vi "Write.vi"(8 "error in (no error)":errorcluster, 10 "Value":sgl, 11 "Local Bus_DBL in":refnum<class "Local Bus_SGL.lvclass">) -> (0 "error out":errorcluster, 3 "Local Bus_DBL out":refnum<class "Local Bus_SGL.lvclass">)   [LabVIEW 2021, in "Local Bus_SGL.lvclass"]
uses:
  Local Bus_SGL.lvclass
  Local Bus_SGL.lvclass/Local Bus_SGL.ctl
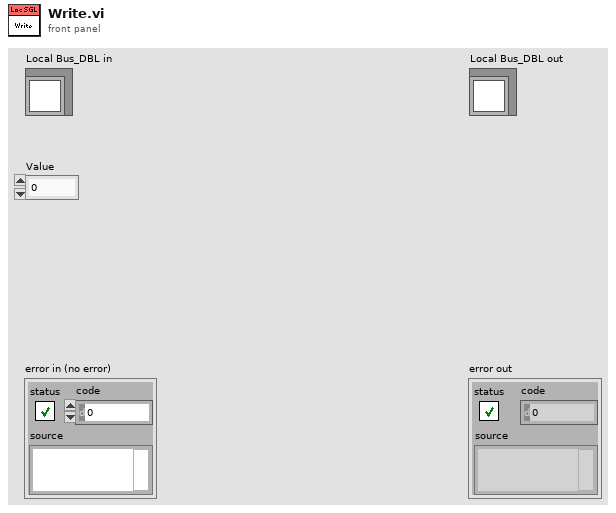
[diagram p1: front panel]
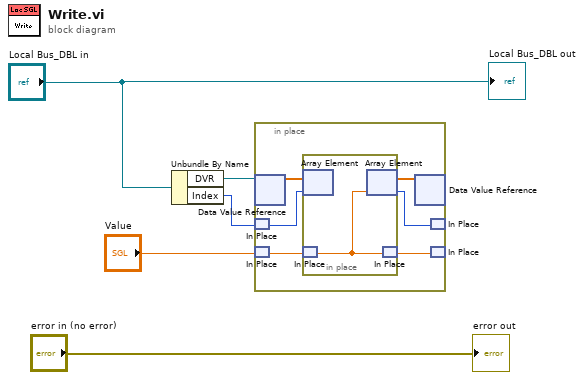
[diagram p0: block diagram]
diagram:
  n1 = Unbundle By Name("Local Bus_DBL in") -> ("DVR"=w4:refnum<data-value>, "Index"=w1:i32)
  n2 = in-place {
    n3 = in-place-dvr #1(w4) -> (w11:sgl[])  [unwired: 1 out]
    n4 = in-place-match #2(w1) -> (w7:i32)
    n5 = in-place-match #3("Value") -> (w9:sgl)
    n6 = in-place {
      n7 = in-place-array #4(w11, w7) -> ()  [unwired: 1 out]
      n8 = in-place-match #5(w9) -> (w12:sgl)
      n9 = in-place-array #4(w12) -> (w10:sgl[], w6:i32)
      n10 = in-place-match #5(w12) -> (w8:sgl)
    }
    n11 = in-place-dvr #1(w10) -> ()  [unwired: 2 out]
    n12 = in-place-match #2(w6) -> ()  [unwired: 1 out]
    n13 = in-place-match #3(w8) -> ()  [unwired: 1 out]
  }
  "error out" <- "error in (no error)"
  "Local Bus_DBL out" <- "Local Bus_DBL in"
